vi "MIO Get QCurve.vi"(1 "Lower Limit":sgl format="%.2f", 2 "Upper Limit":sgl format="%.2f", 3 "Num Sweeps":i32=1) -> (0 "Waveform Graph":dbl[](graph))   [LabVIEW 2009]
uses:
  <vilib>/Daq/zadvd.llb/AO Buffer Write (scaled array).vi
  QCA Global.vi
  <vilib>/Daq/Ai.llb/AI Read (scaled array).vi
panel:
  out "Tune":dbl(slide) scale=-1.0..1.0 scale format="%.2f"
  out "Triangle Wave":dbl[](graph)=[-1.0, -0.996, -0.992, -0.988, -0.984, -0.98, -0.976, -0.972, -0.968, -0.964, -0.96, -0.956, -0.952, -0.948, -0.944, -0.94, -0.9359999999999999, -0.9319999999999999, -0.928, -0.924, -0.92, -0.916, -0.912, -0.908, -0.904, -0.9, -0.896, -0.892, -0.888, -0.884, -0.88, -0.876, -0.872, -0.868, -0.864, -0.86, -0.856, -0.852, -0.848, -0.844, -0.84, -0.836, -0.832, -0.8280000000000001, -0.8240000000000001, -0.8200000000000001, -0.8160000000000001, -0.812, -0.808, -0.804, -0.8, -0.796, -0.792, -0.788, -0.784, -0.78, -0.776, -0.772, -0.768, -0.764, -0.76, -0.756, -0.752, -0.748, -0.744, -0.74, -0.736, -0.732, -0.728, -0.724, -0.72, -0.716, -0.712, -0.708, -0.704, -0.7, -0.696, -0.692, -0.688, -0.6839999999999999, -0.6799999999999999, -0.6759999999999999, -0.6719999999999999, -0.6679999999999999, -0.6639999999999999, -0.6599999999999999, -0.656, -0.652, -0.648, -0.644, -0.64, -0.636, -0.632, -0.628, -0.624, -0.62, -0.616, -0.612, -0.608, -0.604, -0.6, -0.596, -0.5920000000000001, -0.5880000000000001, -0.5840000000000001, -0.5800000000000001, -0.5760000000000001, -0.5720000000000001, -0.5680000000000001, -0.5640000000000001, -0.56, -0.556, -0.552, -0.548, -0.544, -0.54, -0.536, -0.532, -0.528, -0.524, -0.52, -0.516, -0.512, -0.508, -0.504, -0.5, -0.496, -0.492, -0.488, -0.484, -0.48, -0.476, -0.472, -0.46799999999999997, -0.46399999999999997, -0.45999999999999996, -0.45599999999999996, -0.45199999999999996, -0.44799999999999995, -0.44399999999999995, -0.43999999999999995, -0.43600000000000005, -0.43200000000000005, -0.42800000000000005, -0.42400000000000004, -0.42000000000000004, -0.41600000000000004, -0.41200000000000003, -0.40800000000000003, -0.404, -0.4, -0.396, -0.392, -0.388, -0.384, -0.38, -0.376, -0.372, -0.368, -0.364, -0.36, -0.356, -0.352, -0.348, -0.344, -0.33999999999999997, -0.33599999999999997, -0.33199999999999996, -0.32799999999999996, -0.32399999999999995, -0.31999999999999995, -0.31599999999999995, -0.31200000000000006, -0.30800000000000005, -0.30400000000000005, -0.30000000000000004, -0.29600000000000004, -0.29200000000000004, -0.28800000000000003, -0.28400000000000003, -0.28, -0.276, -0.272, -0.268, -0.264, -0.26, -0.256, -0.252, -0.248, -0.244, -0.24, -0.236, -0.23199999999999998, -0.22799999999999998, -0.22399999999999998, -0.21999999999999997, -0.21599999999999997, -0.21199999999999997, -0.20799999999999996, -0.20399999999999996, -0.19999999999999996, -0.19599999999999995, -0.19199999999999995, -0.18799999999999994, -0.18400000000000005, -0.18000000000000005, -0.17600000000000005, -0.17200000000000004, -0.16800000000000004, -0.16400000000000003, -0.16000000000000003, -0.15600000000000003, -0.15200000000000002, -0.14800000000000002, -0.14400000000000002, -0.14, -0.136, -0.132, -0.128, -0.124, -0.12, -0.11599999999999999, -0.11199999999999999, -0.10799999999999998, -0.10399999999999998, -0.09999999999999998, -0.09599999999999997, -0.09199999999999997, -0.08799999999999997, -0.08399999999999996, -0.07999999999999996, -0.07599999999999996, -0.07199999999999995, -0.06799999999999995, -0.06399999999999995, -0.06000000000000005, -0.05600000000000005, -0.052000000000000046, -0.04800000000000004, -0.04400000000000004, -0.040000000000000036, -0.03600000000000003, -0.03200000000000003, -0.028000000000000025, -0.02400000000000002, -0.020000000000000018, -0.016000000000000014, -0.01200000000000001, -0.008000000000000007, -0.0040000000000000036, 0.0, 0.0040000000000000036, 0.008000000000000007, 0.01200000000000001, 0.016000000000000014, 0.020000000000000018, 0.02400000000000002, 0.028000000000000025, 0.03200000000000003, 0.03600000000000003, 0.040000000000000036, 0.04400000000000004, 0.04800000000000004, 0.052000000000000046, 0.05600000000000005, 0.06000000000000005, 0.06400000000000006, 0.06800000000000006, 0.07200000000000006, 0.07600000000000007, 0.08000000000000007, 0.08400000000000007, 0.08800000000000008, 0.09200000000000008, 0.09600000000000009, 0.10000000000000009, 0.10400000000000009, 0.1080000000000001, 0.1120000000000001, 0.1160000000000001, 0.1200000000000001, 0.12400000000000011, 0.1279999999999999, 0.1319999999999999, 0.1359999999999999, 0.1399999999999999, 0.1439999999999999, 0.1479999999999999, 0.1519999999999999, 0.15599999999999992, 0.15999999999999992, 0.16399999999999992, 0.16799999999999993, 0.17199999999999993, 0.17599999999999993, 0.17999999999999994, 0.18399999999999994, 0.18799999999999994, 0.19199999999999995, 0.19599999999999995, 0.19999999999999996, 0.20399999999999996, 0.20799999999999996, 0.21199999999999997, 0.21599999999999997, 0.21999999999999997, 0.22399999999999998, 0.22799999999999998, 0.23199999999999998, 0.236, 0.24, 0.244, 0.248, 0.252, 0.256, 0.26, 0.264, 0.268, 0.272, 0.276, 0.28, 0.28400000000000003, 0.28800000000000003, 0.29200000000000004, 0.29600000000000004, 0.30000000000000004, 0.30400000000000005, 0.30800000000000005, 0.31200000000000006, 0.31600000000000006, 0.32000000000000006, 0.32400000000000007, 0.32800000000000007, 0.3320000000000001, 0.3360000000000001, 0.3400000000000001, 0.3440000000000001, 0.3480000000000001, 0.3520000000000001, 0.3560000000000001, 0.3600000000000001, 0.3640000000000001, 0.3680000000000001, 0.3720000000000001, 0.3759999999999999, 0.3799999999999999, 0.3839999999999999, 0.3879999999999999, 0.3919999999999999, 0.3959999999999999, 0.3999999999999999, 0.4039999999999999, 0.4079999999999999, 0.4119999999999999, 0.4159999999999999, 0.41999999999999993, 0.42399999999999993, 0.42799999999999994, 0.43199999999999994, 0.43599999999999994, 0.43999999999999995, 0.44399999999999995, 0.44799999999999995, 0.45199999999999996, 0.45599999999999996, 0.45999999999999996, 0.46399999999999997, 0.46799999999999997, 0.472, 0.476, 0.48, 0.484, 0.488, 0.492, 0.496, 0.5, 0.504, 0.508, 0.512, 0.516, 0.52, 0.524, 0.528, 0.532, 0.536, 0.54, 0.544, 0.548, 0.552, 0.556, 0.56, 0.5640000000000001, 0.5680000000000001, 0.5720000000000001, 0.5760000000000001, 0.5800000000000001, 0.5840000000000001, 0.5880000000000001, 0.5920000000000001, 0.5960000000000001, 0.6000000000000001, 0.6040000000000001, 0.6080000000000001, 0.6120000000000001, 0.6160000000000001, 0.6200000000000001, 0.6240000000000001, 0.6279999999999999, 0.6319999999999999, 0.6359999999999999, 0.6399999999999999, 0.6439999999999999, 0.6479999999999999, 0.6519999999999999, 0.6559999999999999, 0.6599999999999999, 0.6639999999999999, 0.6679999999999999, 0.6719999999999999, 0.6759999999999999, 0.6799999999999999, 0.6839999999999999, 0.688, 0.692, 0.696, 0.7, 0.704, 0.708, 0.712, 0.716, 0.72, 0.724, 0.728, 0.732, 0.736, 0.74, 0.744, 0.748, 0.752, 0.756, 0.76, 0.764, 0.768, 0.772, 0.776, 0.78, 0.784, 0.788, 0.792, 0.796, 0.8, 0.804, 0.808, 0.812, 0.8160000000000001, 0.8200000000000001, 0.8240000000000001, 0.8280000000000001, 0.8320000000000001, 0.8360000000000001, 0.8400000000000001, 0.8440000000000001, 0.8480000000000001, 0.8520000000000001, 0.8560000000000001, 0.8600000000000001, 0.8640000000000001, 0.8680000000000001, 0.8720000000000001, 0.8759999999999999, 0.8799999999999999, 0.8839999999999999, 0.8879999999999999, 0.8919999999999999, 0.8959999999999999, 0.8999999999999999, 0.9039999999999999, 0.9079999999999999, 0.9119999999999999, 0.9159999999999999, 0.9199999999999999, 0.9239999999999999, 0.9279999999999999, 0.9319999999999999, 0.9359999999999999, 0.94, 0.944, 0.948, 0.952, 0.956, 0.96, 0.964, 0.968, 0.972, 0.976, 0.98, 0.984, 0.988, 0.992, 0.996]
  # "A\nD\nD\n\nP\nH\nA\nS\nE"
  # "R\nE\nM\nO\nV\nE\n\nP\nH\nA\nS\nE"
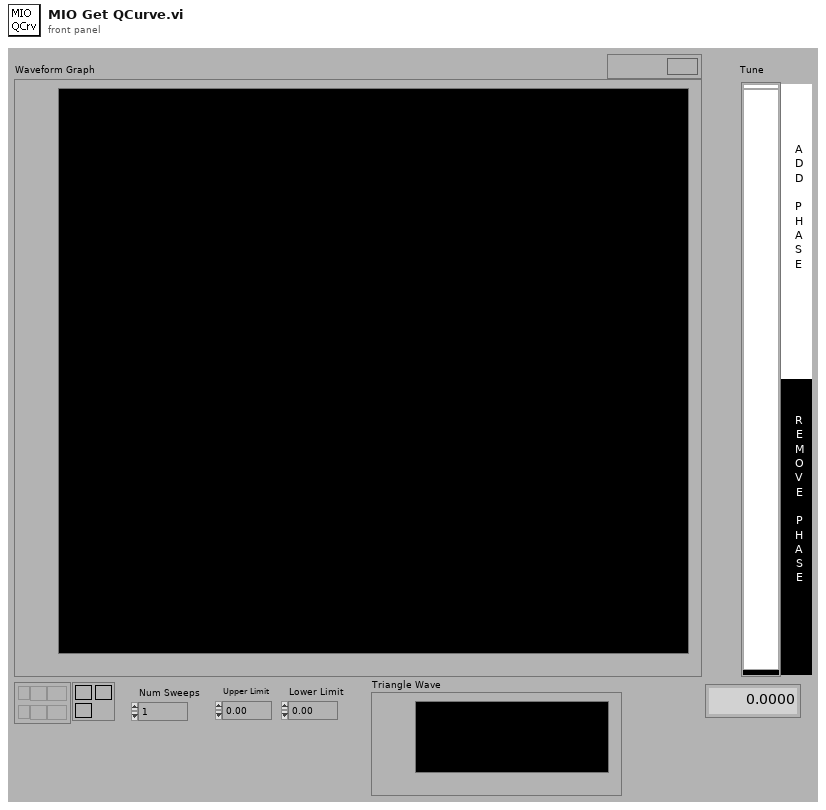
[diagram p1: front panel]
types:
  T1 = cluster{"upper limit (V)":sgl, "lower limit (V)":sgl, "reference source":enum16{"no change", "internal", "external"}}[]
  T2 = enum16{"ungated/software start", "count while high", "count while low", "start on rising edge", "start on falling edge", "restart on each rising edge", "restart on each falling edge"}
  T3 = enum16{"no change", "none", "trigger on rising edge", "trigger on falling edge", "pause while gate is TTL high", "pause while gate is TTL low"}
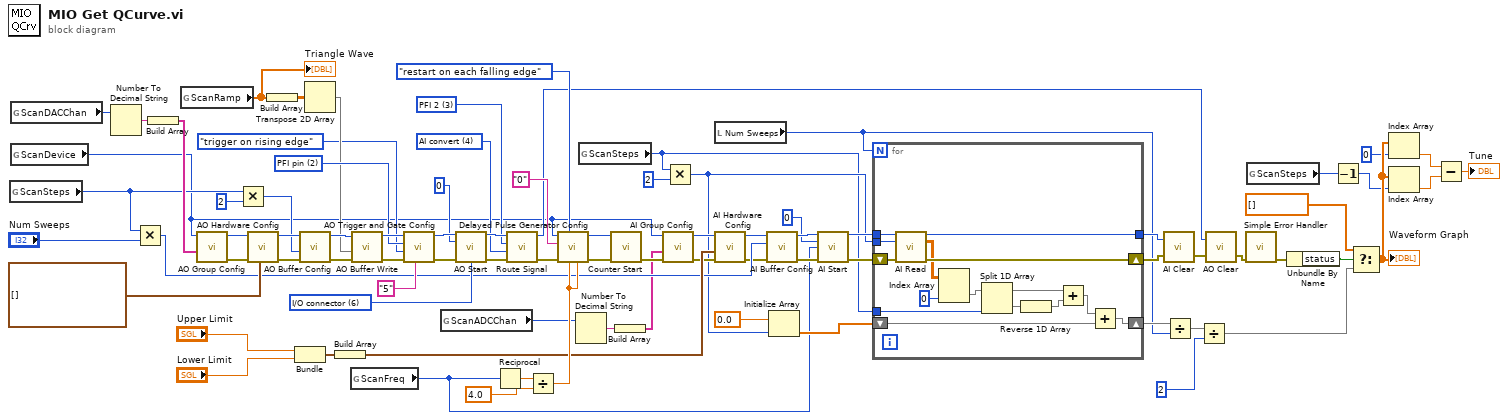
[diagram p0: block diagram]
diagram:
  w64 = u16 4 items=["no change", "none", "AI start trigger", "AI stop trigger", "AI convert", "GPCTR 1 source", "GPCTR 1 gate", "AO update", "AO start trigger", "AI scan start", "GPCTR  0 source", "GPCTR  0 gate", "GPCTR  0 output", "RTSI 0", "RTSI 1", "RTSI 2", "RTSI 3", "RTSI 4", "RTSI 5", "RTSI 6", "RTSI clock", "board clock", "PLL input pin", "marker out", "SYNC out", "analog trigger circuit output", "end of acquisition", "frequency output", "high", "low", "SCANCLK", "inverted voltmeter complete", "voltmeter complete", "GPCTR n source", "GPCTR n gate", "GPCTR n output", "PFI n", "AI scan in progress", "(Reserved_1)", "(Reserved_2)", "stable 10MHz"] ("signal source")
  w65 = u16 3 items=["no change", "PFI 0", "PFI 1", "PFI 2", "PFI 3", "PFI 4", "PFI 5", "PFI 6", "PFI 7", "PFI 8", "PFI 9", "GPCTR 0 output", "RTSI 0", "RTSI 1", "RTSI 2", "RTSI 3", "RTSI 4", "RTSI 5", "RTSI 6", "RTSI clock", "board clock", "PLL reference clock", "SCANCLK", "I/O connector", "PFI n", "start trigger", "configurable filter", "PXI backplane clock"] ("signal name")
  w66 = u16 6 items=["no change", "internal", "counter 1", "counter 2", "counter 3", "counter 5", "I/O connector", "RTSI connection", "PFI pin, low to high", "PFI pin, high to low", "RTSI pin, low to high", "RTSI pin, high to low", "GPCTR 1 output, low to high", "GPCTR 1 output, high to low", "ATCOUT, low to high", "ACTOUT, high to low", "internal clock 2"] ("clock source (internal:1)")
  w68 = u16 2 items=["no change", "none", "PFI pin", "RTSI pin", "AI start trigger", "ATCOUT", "trigger input connector"] ("trigger or gate source (0: no change)")
  n1 = global read "QCA Global.vi" "ScanSteps"() -> (w6:i32)
  n2 = global read "QCA Global.vi" "ScanDACChan"() -> (w7:i32)
  n3 = global read "QCA Global.vi" "ScanDevice"() -> (w5:i32)
  n4 = Number To Decimal String(number=w7) -> (decimal integer string=w24:string)  [unwired: 1 in]
  n5 = Multiply(x=w6, y="Num Sweeps") -> (x*y=w42:i32)
  n6 = Build Array(w24) -> (w23:string[])
  n7 = global read "QCA Global.vi" "ScanRamp"() -> (w28:dbl[])
  "Triangle Wave" <- w28
  n8 = call <vilib>:"AO Group Config.vi"("channel list (empty)"=w23, "device"=w5) -> ("error out"=w60:errorcluster, "task ID out"=w75:u32)  [unwired: 7 in, 1 out]
  n9 = Multiply(x=w6, y=2) -> (x*y=w51:i32)
  n10 = call <vilib>:"AO Hardware Config.vi"("limit settings (no change)"=T1 [], "error in (no error)"=w60, "task ID"=w75) -> ("error out"=w83:errorcluster, "task ID out"=w74:u32)  [unwired: 6 in, 1 out]
  n11 = Build Array(w28) -> (w54:dbl[][])
  n12 = Bundle("Upper Limit"="Upper Limit", "Lower Limit"="Lower Limit") -> (w50:cluster{"Upper Limit":sgl, "Lower Limit":sgl})  [unwired: 1 in]
  n13 = call <vilib>:"AO Buffer Config.vi"("error in (no error)"=w83, "number of updates\n (-1: no change)"=w51, "task ID"=w74) -> ("error out"=w58:errorcluster, "task ID out"=w73:u32)  [unwired: 7 in]
  n14 = Transpose 2D Array(2D array=w54) -> (transposed array=w53:dbl[][])
  n15 = Build Array(w50) -> (w46:cluster{"Upper Limit":sgl, "Lower Limit":sgl}[])
  n16 = global read "QCA Global.vi" "ScanFreq"() -> (w3:i32)
  n17 = call-poly <vilib>:"AO Buffer Write.vi"("error in (no error)"=w58, "scaled data (empty)"=w53, "task ID"=w73) -> ("error out"=w59:errorcluster, "task ID out"=w72:u32)  [unwired: 6 in, 1 out]
  n18 = call <vilib>:"AO Trigger and Gate Config.vi"("trigger or gate  source specification"="5", "error in (no error)"=w59, "trigger or gate condition (0: no change)"=T3."trigger on rising edge", "trigger or gate source (0: no change)"=w68, "task ID"=w72) -> ("error out"=w77:errorcluster, "task ID out"=w71:u32)  [unwired: 5 in]
  n19 = global read "QCA Global.vi" "ScanADCChan"() -> (w4:i32)
  n20 = call <vilib>:"AO Start.vi"("taskID in"=w71, "number of buffer iterations (1)"=0, "error in (no error)"=w77, "clock source (internal:1)"=w66) -> ("taskID out"=w69:u32, "error out"=w82:errorcluster)  [unwired: 9 in, 1 out]
  n21 = Reciprocal(x=w3) -> (1/x=w56:dbl)
  n22 = call <vilib>:"Route Signal.vi"("error in (no error)"=w82, "signal source"=w64, "signal name"=w65, "task ID"=w69) -> ("error out"=w81:errorcluster, "task ID out"=w61:u32)  [unwired: 6 in]
  n23 = Divide(x=w56, y=sgl 4.0 ("Input")) -> (x/y=w57:dbl)
  n24 = call <vilib>:"Delayed Pulse Generator Config.vi"("pulse width (s or cycles)"=w57, "pulse delay (s or cycles)"=w57, "gate mode (ungated:0)"=T2."restart on each falling edge", "error in (no error)"=w81, "counter"="0", "device"=w5) -> ("error out"=w80:errorcluster, "taskID"=w70:u32)  [unwired: 2 in, 2 out]
  n25 = Number To Decimal String(number=w4) -> (decimal integer string=w26:string)  [unwired: 1 in]
  n26 = global read "QCA Global.vi" "ScanSteps"() -> (w1:i32)
  n27 = call <vilib>:"Counter Start.vi"("error in (no error)"=w80, "taskID"=w70) -> ("error out"=w79:errorcluster)  [unwired: 8 in, 1 out]
  n28 = Build Array(w26) -> (w25:string[])
  n29 = call <vilib>:"AI Group Config.vi"("error in (no error)"=w79, "channel scan list (empty)"=w25, "device"=w5) -> ("error out"=w39:errorcluster, "task ID"=w38:u32)  [unwired: 6 in, 1 out]
  n30 = Multiply(x=w1, y=2) -> (x*y=w29:i32)
  n31 = local read "Num Sweeps"() -> (w18:i32)
  n32 = call <vilib>:"AI Hardware Config.vi"("error in (no error)"=w39, "input limits(no change)"=w46, "task ID"=w38) -> ("error out"=w41:errorcluster, "task ID out"=w37:u32)  [unwired: 6 in, 1 out]
  n33 = call <vilib>:"AI Buffer Config.vi"("error in (no error)"=w41, "scans per buffer (-1: no change)"=w42, "task ID"=w37) -> ("error out"=w40:errorcluster, "task ID out"=w36:u32)  [unwired: 7 in]
  n34 = Initialize Array(sgl 0.0 ("Element Data"), w29) -> (w33:sgl[])
  n35 = call <vilib>:"AI Start.vi"("taskID in"=w36, "number of scans to acquire (-1)"=0, "scan rate (1000 scans/sec)"=w3, "error in (no error)"=w40) -> ("taskID out"=w31:u32, "error out"=w30:errorcluster)  [unwired: 8 in, 2 out]
  n36 = for {
    N: w18 -> [_]
    tunnel: w29 -> [w98]
    shift-right: [w96] -> w43
    shift-left: w30 -> [w97]
    tunnel: w31 -> [w95]
    tunnel: [w94] -> w44
    tunnel: w1 -> [w88]
    shift-right: [w86] -> w19
    shift-left: w33 -> [w87]
    n37 = call-poly <vilib>:"AI Read.vi"("taskID in"=w95, "number of scans to read (-1:all)"=w98, "error in (no error)"=w97) -> ("taskID out"=w94:u32, "scaled data"=w89:sgl[][], "error out"=w96:errorcluster)  [unwired: 7 in, 3 out]
    n38 = Index Array(array=w89, index (col)=0 ("Index")) -> (element=w85:sgl[])  [unwired: 1 in]
    n39 = Split 1D Array(array=w85, index=w88) -> (first subarray=w93:sgl[], second subarray=w91:sgl[])
    n40 = Reverse 1D Array(array=w91) -> (reversed array=w92:sgl[])
    n41 = Add(x=w93, y=w92) -> (x+y=w84:sgl[])
    n42 = Add(x=w84, y=w87) -> (x+y=w86:sgl[])
  }
  n43 = call <vilib>:"AI Clear.vi"("error in (no error)"=w43, "taskID in"=w44) -> ("error out"=w45:errorcluster)  [unwired: 4 in, 1 out]
  n44 = Divide(x=w19, y=w18) -> (x/y=w17:sgl[])
  n45 = Divide(x=w17, y=2) -> (x/y=w15:sgl[])
  n46 = call <vilib>:"AO Clear.vi"("error in (no error)"=w45, "taskID in"=w61) -> ("error out"=w78:errorcluster)  [unwired: 4 in, 1 out]
  n47 = call <vilib>:"Simple Error Handler.vi"("error in (no error)"=w78) -> ("error out"=w21:errorcluster)  [unwired: 4 in, 4 out]
  n48 = global read "QCA Global.vi" "ScanSteps"() -> (w2:i32)
  n49 = Unbundle By Name(w21) -> ("status"=w20:bool)
  n50 = Decrement(x=w2) -> (x-1=w9:i32)
  n51 = Select(t=dbl[] [], s=w20, f=w15) -> (s? t:f=w11:dbl[])
  "Waveform Graph" <- w11
  n52 = Index Array(array=w11, index=0 ("Index")) -> (element=w12:dbl)
  n53 = Index Array(array=w11, index=w9) -> (element=w13:dbl)
  n54 = Subtract(x=w12, y=w13) -> (x-y=→"Tune":dbl)
